vi "Setup.vi"(8 "error in (no error)":errorcluster, 11 "Process Test In":refnum<class "Person Test.lvclass">) -> (0 "error out":errorcluster, 3 "Process Test Out":refnum<class "Person Test.lvclass">)   [LabVIEW 2020, in "Person Test.lvclass"]
uses:
  Person Test.lvclass
  C:/Program Files (x86)/National Instruments/LabVIEW 2020/vi.lib/Asteme/Triarc Framework Test Suite/Base Class Test/Base Test.lvclass
  Person/Person.lvclass
  C:/Program Files (x86)/National Instruments/LabVIEW 2020/vi.lib/Asteme/Triarc Framework/Base/Base.lvclass
  <vilib>/Asteme/Triarc Framework Test Suite/Base Class Test/Base Test.lvclass/Base Test.ctl
  <vilib>/Asteme/Triarc Framework Test Suite/Base Class Test/Base Test.lvclass
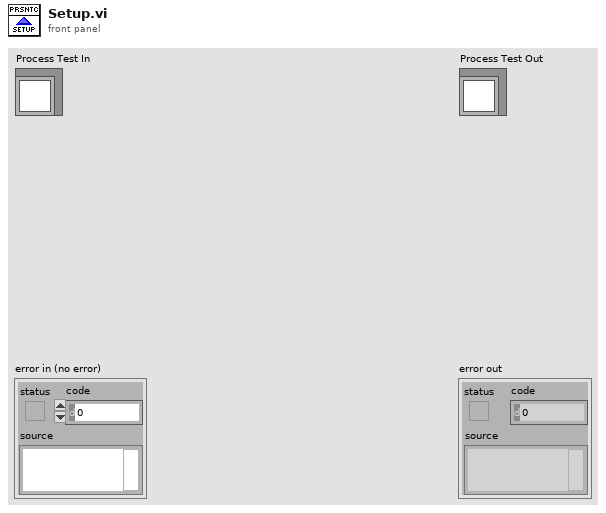
[diagram p1: front panel]
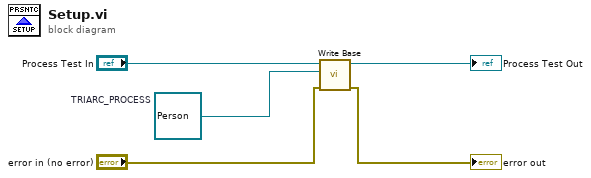
[diagram p0: block diagram]
diagram:
  w3 = refnum<class "Person.lvclass"> refnum  # TRIARC_PROCESS
  n1 = call <vilib>:"Write Base.vi"("error in (no error)"="error in (no error)", "Base"=w3, "Base Class Test In"="Process Test In") -> ("error out"=→"error out":errorcluster, "Base Class Test Out"=→"Process Test Out":refnum<class "Person Test.lvclass">)  [unwired: 7 in]
